vi "Lock.vi"(8 "error in (no error)":errorcluster, 11 "Door in":refnum<class "Door.lvclass">) -> (0 "error out":errorcluster, 3 "Door out":refnum<class "Door.lvclass">)   [LabVIEW 2018, in "Door.lvclass"]
uses:
  Door.lvclass
  Door.lvclass/Door.ctl
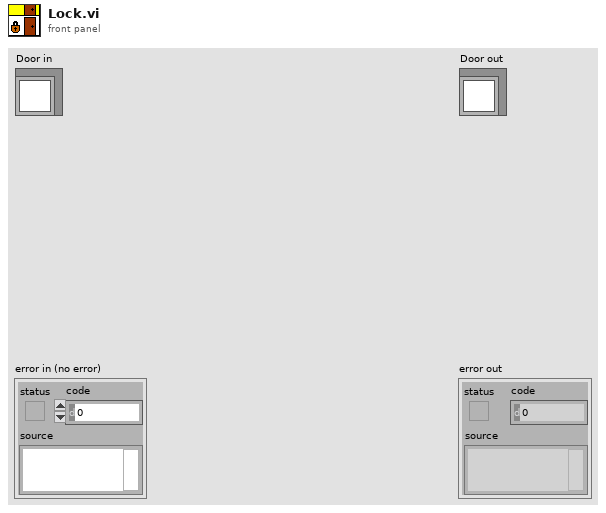
[diagram p1: front panel]
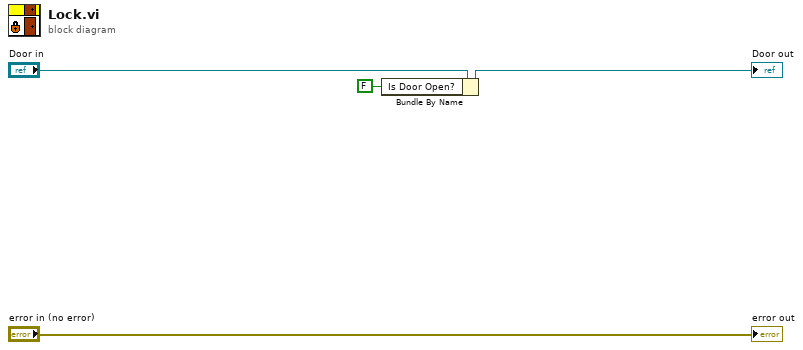
[diagram p0: block diagram]
diagram:
  n1 = Bundle By Name(cluster="Door in", "Is Door Open?"=FALSE) -> (→"Door out":refnum<class "Door.lvclass">)
  "error out" <- "error in (no error)"
